vi "generate_unique_pulsed_filename.vi"(10 "Filename (no extension)":string, 11 "Data Folder":path) -> (2 "Filename":path)   [LabVIEW 2016]
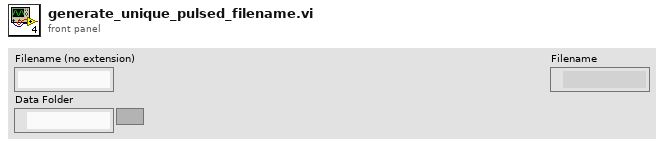
[diagram p1: front panel]
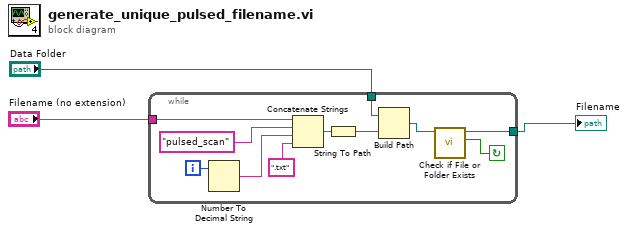
[diagram p0: block diagram]
diagram:
  n1 = while {
    tunnel: "Filename (no extension)" -> [w14]
    tunnel: [w7] -> w2
    tunnel: "Data Folder" -> [w4]
    i -> [w12]
    stop <- w8 continue-if-true
    n2 = Number To Decimal String(number=w12) -> (decimal integer string=w11:string)  [unwired: 1 in]
    n3 = Concatenate Strings(w14, "pulsed_scan", w11, ".txt") -> (w9:string)
    n4 = String To Path(string=w9) -> (path=w6:path)
    n5 = Build Path(base path=w4, name or relative path=w6) -> (appended path=w5:path)
    n6 = call <vilib>:"Check if File or Folder Exists.vi"("path"=w5) -> ("file or folder exists?"=w8:bool, "dup path"=w7:path)  [unwired: 8 in, 1 out]
  }
  "Filename" <- w2
